vi "uMsg_Delayed Abort future copies.vi"(8 "error in (no error)":errorcluster, 11 "uMsg_Delayed in":refnum<class "uMsg_Delayed.lvclass">) -> (0 "error out":errorcluster)   [LabVIEW 2023, in "uLib.lvlib" / "uMsg_Delayed.lvclass"]
doc: "Invoke this method to abort the any future pending messages. None of the scheduled copies will be processed.\n\nThis method executed regardless of the error state."
uses:
  uMsg_Delayed.lvclass
  uMsg_Delayed.lvclass/uMsg_Delayed.ctl
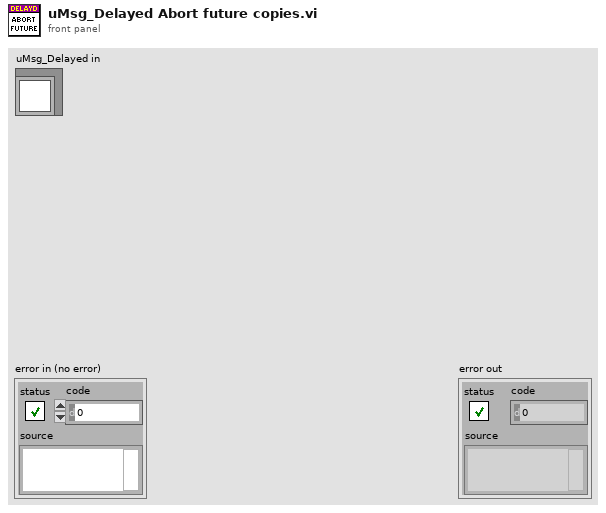
[diagram p1: front panel]
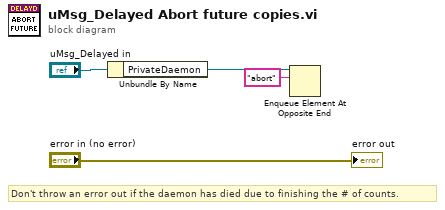
[diagram p0: block diagram]
diagram:
  # "Don't throw an error out if the daemon has died due to finishing the # of counts."
  n1 = Unbundle By Name("uMsg_Delayed in") -> ("PrivateDaemon"=w2:refnum<queue>)
  n2 = Enqueue Element At Opposite End(queue=w2, element="abort") -> ()  [unwired: 2 in, 3 out]
  "error out" <- "error in (no error)"
